vi "1-9.vi"() -> ()   [LabVIEW 2022 SP3]
panel:
  out "数值 3":dbl
  in  "数值 2":dbl
  in  "数值":dbl
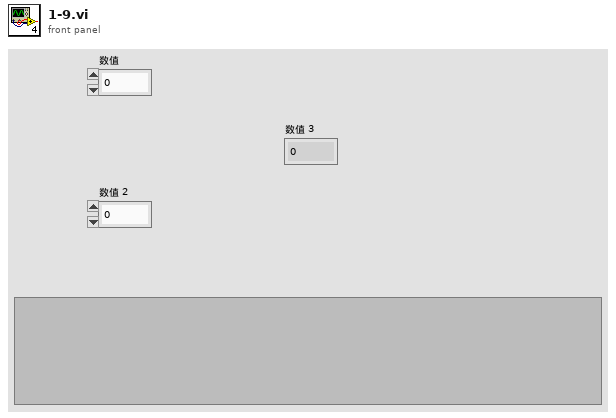
[diagram p1: front panel]
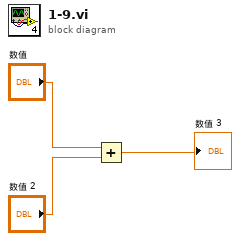
[diagram p0: block diagram]
diagram:
  n1 = Add(x="数值", y="数值 2") -> (x+y=→"数值 3":dbl)
